vi "FindServo_NoWhile.vi"(0 "Amplitude Reference Array":refnum<vi>[](array[refnum]), 1 "Parameter Reference Arrary":refnum<vi>[](array[refnum]), 4 "Length Array":dbl[](array[numeric]), 7 "Parameter Cluster":T1={"Amplitude (cm)"=4.0, "Frequency (Hz)"=1.0, "Number of Waves"=1.0, "Length of MBE (cm)"=10.0, "Wave Exponential"=2.0, "Number of Servos"=5.0, "Bend Amplitude 1"=0.1, "Bend Amplitude 2"=0.2, "Bend Phase 1"=0.0, "Bend Phase 2"=0.8499}, 8 "Wave Form":u16(ring) items=["Sine", "Exponentional Sine", "Two Beam Bending", "Flat Plate"], 10 "2nd Mode Bending Options":u16(ring) items=["Specifiy Tail Amplitude & 1st Mode", "Specifiy Tail Amplitude & 2nd Mode", ""], 12 "Wind Up":bool, 13 "Start Time (Tick Count-millis)":u32, 14 "Wind Down":bool, 15 "Wind Down Time":i32=5, 16 "Stop In":bool, 17 "Stop Pressed Shift In (False)":bool, 19 "Ms Since Stop Shift In (Start Time)":u32, 23 "Stop In Reference":refnum<vi>, 27 "S since stop Shift In":dbl) -> (18 "Stop Out":bool, 20 "phi":dbl[](array[numeric]), 21 "X Nodes":dbl[](array[numeric]), 22 "Y Nodes":dbl[](array[numeric]), 24 "Stop Pressed Shift Out (False)":bool, 25 "MS Since Stop Shift Out":u32, 26 "S since stop Shift Out":dbl)   [LabVIEW 2017]
panel:
  out "Simulation Time":dbl
  # "Off"
  # "On"
  # "Off"
  # "On"
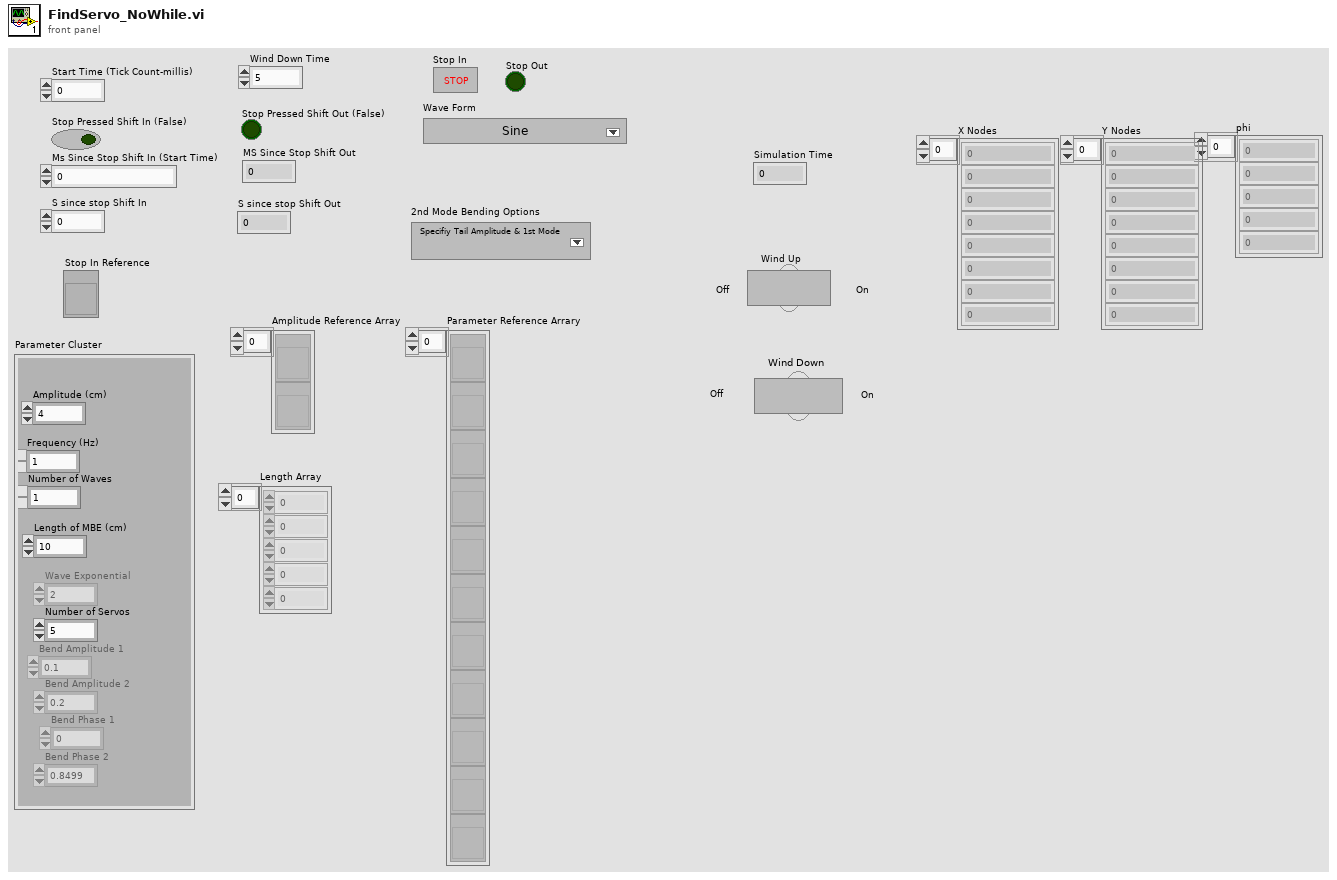
[diagram p1: front panel]
types:
  T1 = cluster{"Amplitude (cm)":dbl, "Frequency (Hz)":dbl, "Number of Waves":dbl, "Length of MBE (cm)":dbl, "Wave Exponential":dbl, "Number of Servos":dbl, "Bend Amplitude 1":dbl, "Bend Amplitude 2":dbl, "Bend Phase 1":dbl, "Bend Phase 2":dbl}
  T2 = enum8{"Enabled", "Disabled", "Disabled and Grayed Out"}
  T3 = enum8{"Enabled", "Disabled", "Disabled and Grayed Out"}[]
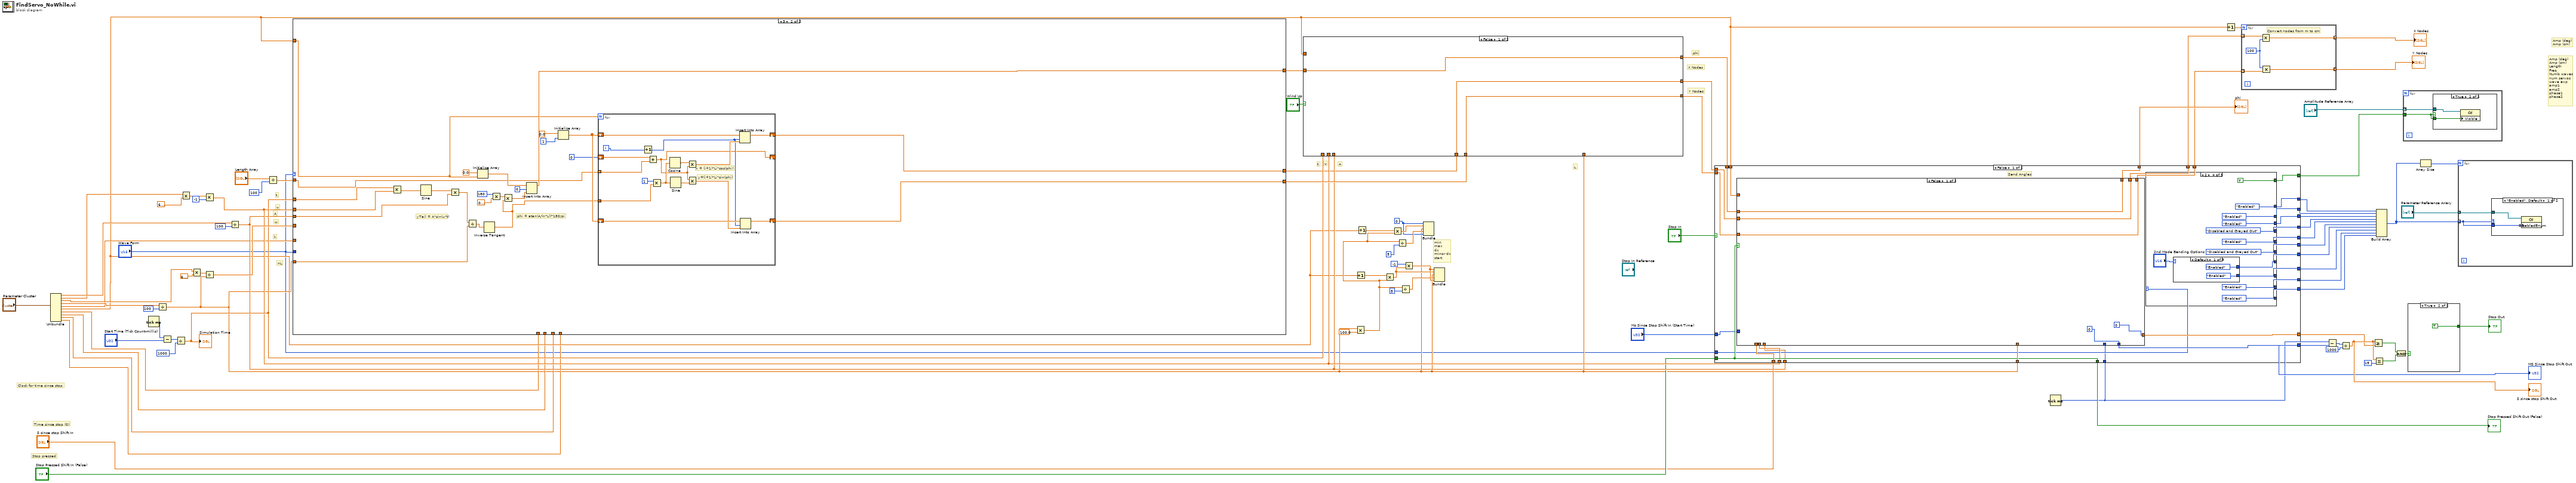
[diagram p0: block diagram]
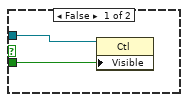
[diagram p2: hidden frame]
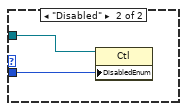
[diagram p3: hidden frame]
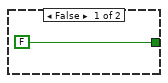
[diagram p4: hidden frame]
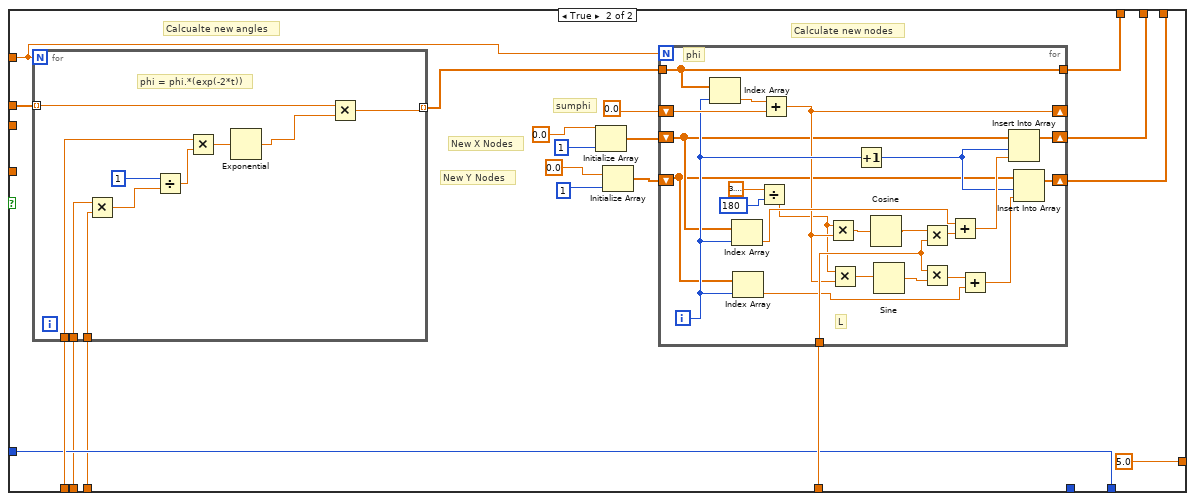
[diagram p5: hidden frame]
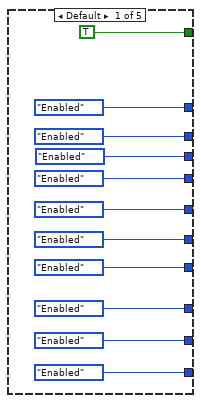
[diagram p6: hidden frame]
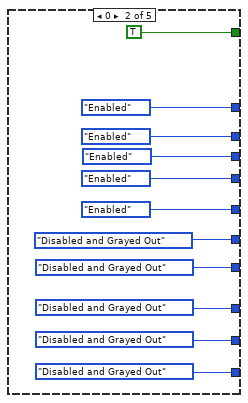
[diagram p7: hidden frame]
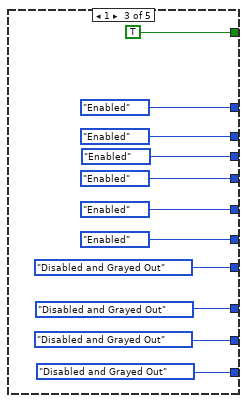
[diagram p8: hidden frame]
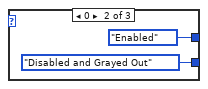
[diagram p9: hidden frame]
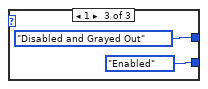
[diagram p10: hidden frame]
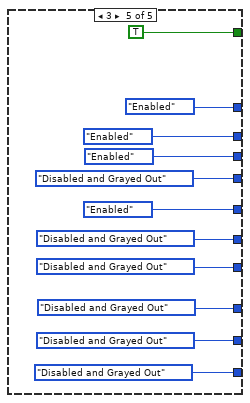
[diagram p11: hidden frame]
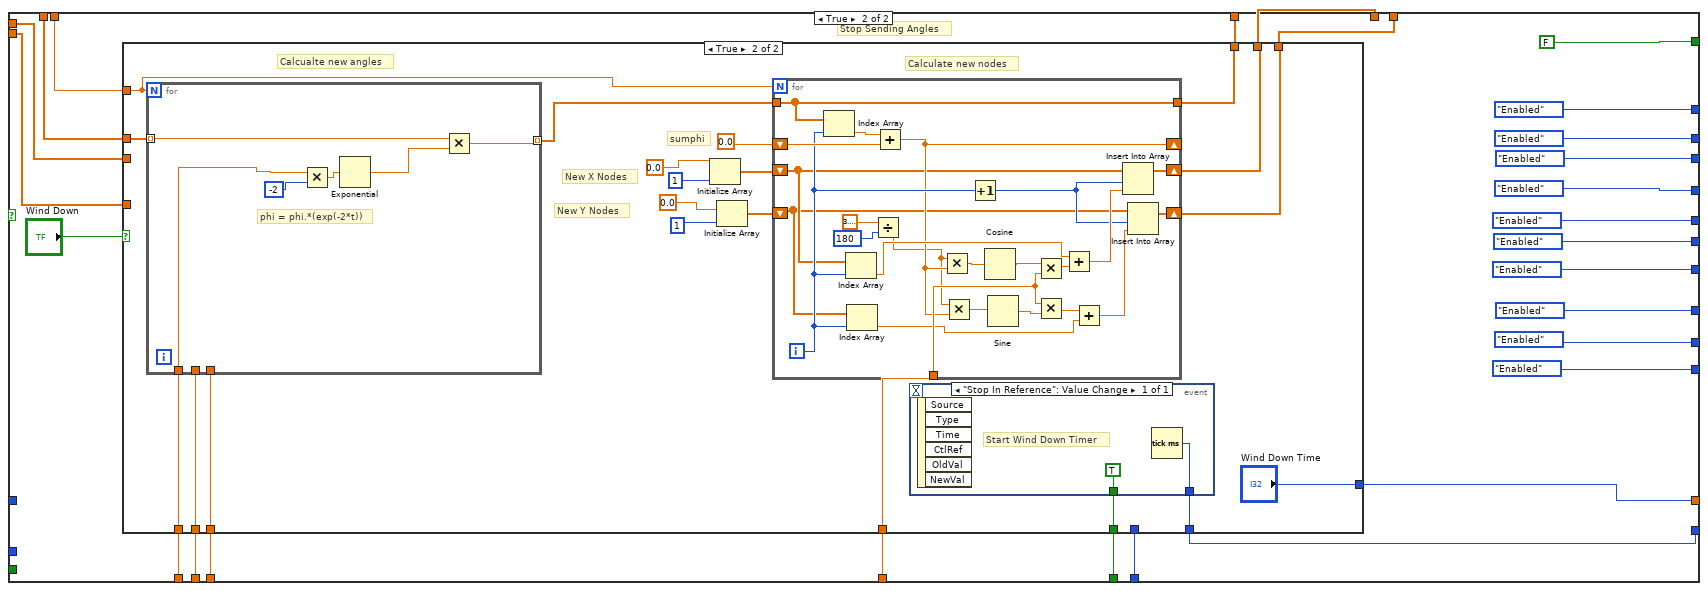
[diagram p12: hidden frame]
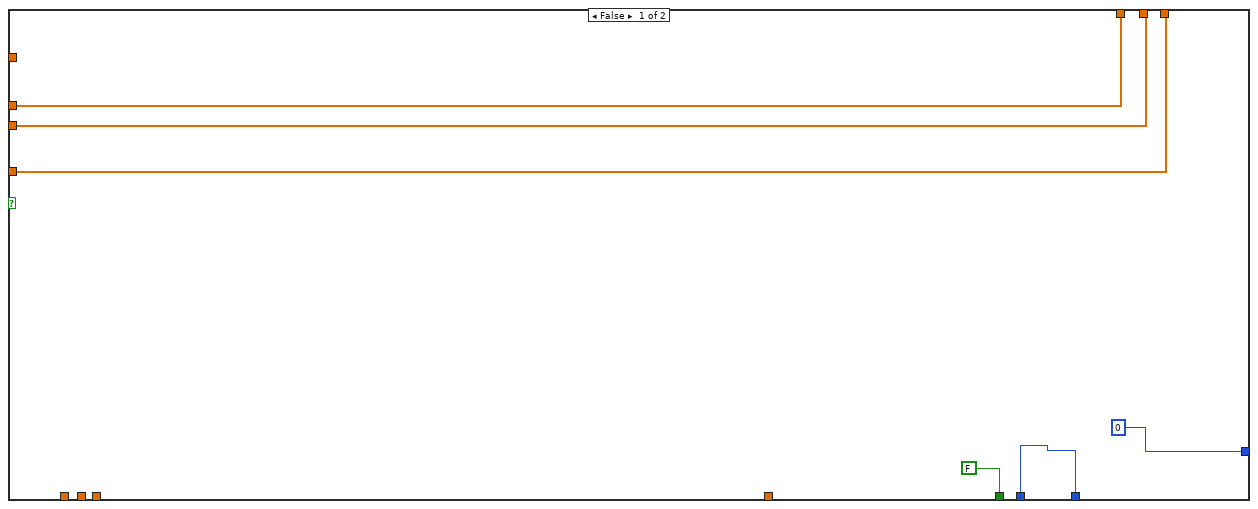
[diagram p13: hidden frame]
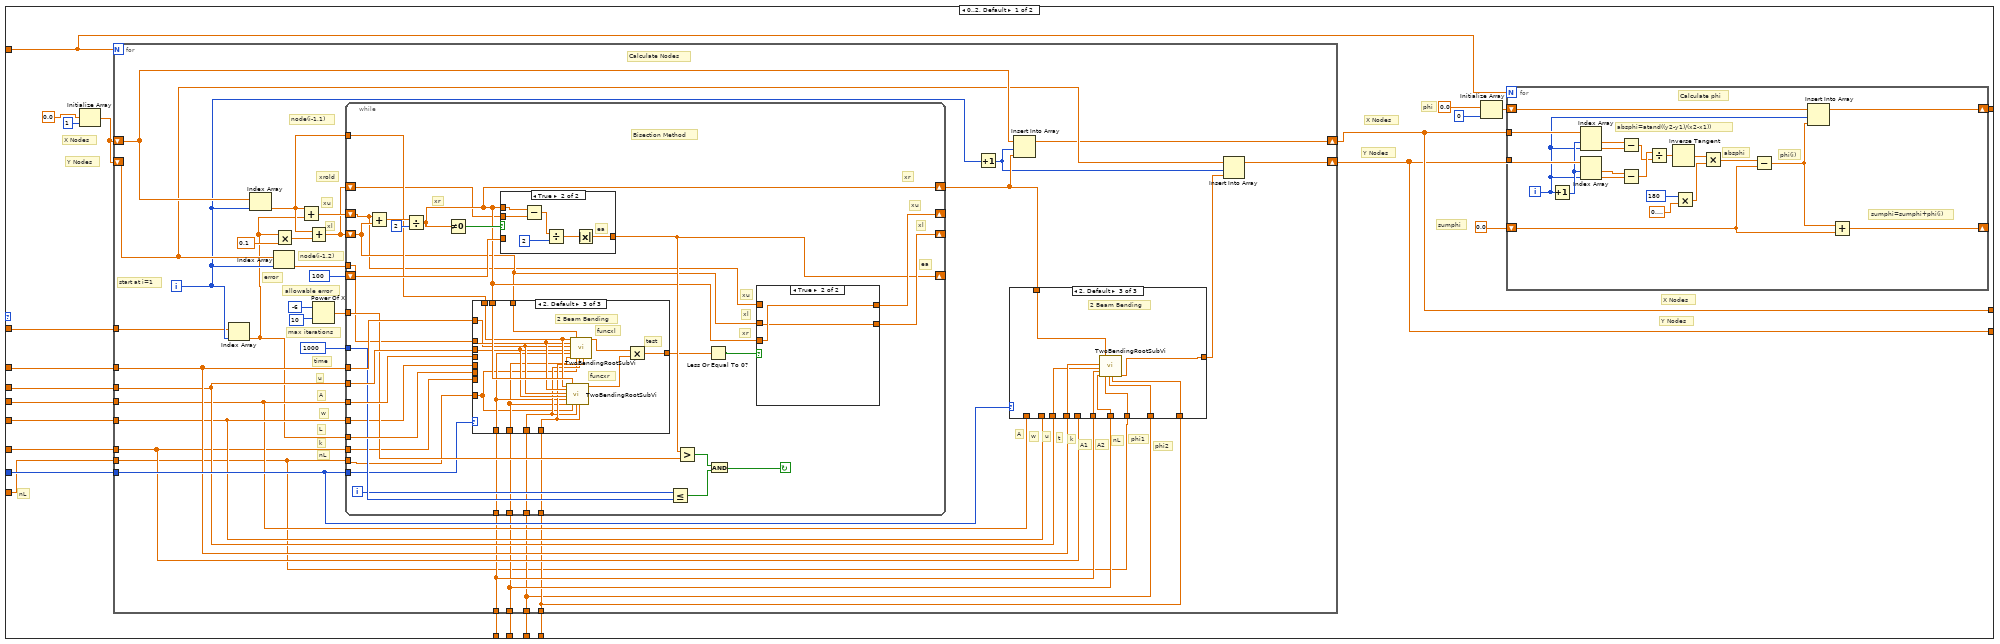
[diagram p14: hidden frame]
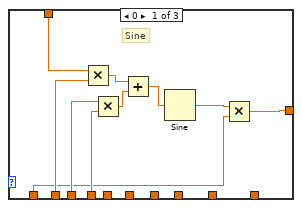
[diagram p15: hidden frame]
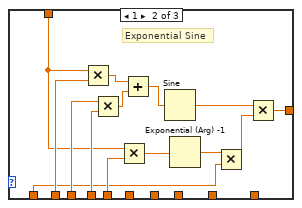
[diagram p16: hidden frame]
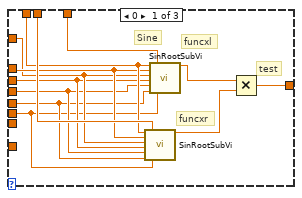
[diagram p19: hidden frame]
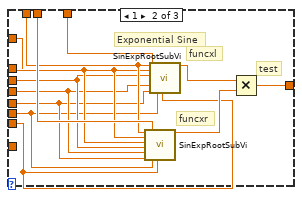
[diagram p20: hidden frame]
diagram:
  w63 = 0
  # "nL"
  # "Amp (deg)\nAmp (cm)"
  # "Amp (deg)\nAmp (cm)\nLength\nFreq\nNumb waves\nnum servos\nwave exp\namp1\namp2\nphase1\nphase2"
  # "Y Nodes"
  # "X Nodes"
  # "phi"
  # "k"
  # "min\nmax\ndx\nminor dx\nstart"
  # "A"
  # "t"
  # "L"
  # "A"
  # "u"
  # "t"
  # "u"
  # "w"
  # "Stop pressed"
  # "Clock for time since stop"
  # "Time since stop (0)"
  n1 = Unbundle("Parameter Cluster") -> ("Amplitude (cm)"=w17:dbl, "Frequency (Hz)"=w16:dbl, "Number of Waves"=w15:dbl, "Length of MBE (cm)"=w14:dbl, "Wave Exponential"=w13:dbl, "Number of Servos"=w12:dbl, "Bend Amplitude 1"=w11:dbl, "Bend Amplitude 2"=w10:dbl, "Bend Phase 1"=w9:dbl, "Bend Phase 2"=w8:dbl)
  n2 = Tick Count (ms)() -> (millisecond timer value=w78:u32)
  n3 = Divide(x=w14, y=100) -> (x/y=w3:dbl)
  n4 = Subtract(x=w78, y="Start Time (Tick Count-millis)") -> (x-y=w77:u32)
  n5 = Divide(x=w77, y=1000) -> (x/y=w59:dbl)
  "Simulation Time" <- w59
  n6 = Multiply(x=w16, y=6.283185307179586) -> (x*y=w83:dbl)
  n7 = Multiply(x=w15, y=6.283185307179586) -> (x*y=w86:dbl)
  n8 = Multiply(x=w83, y=-1) -> (x*y=w58:dbl)
  n9 = Divide(x=w86, y=w3) -> (x/y=w81:dbl)
  n10 = Divide(x=w17, y=100) -> (x/y=w57:dbl)
  n11 = Divide(x="Length Array", y=100) -> (x/y=w4:dbl[])
  n12 = case shown="3" "Wave Form" {
    tunnel: "Wave Form" -> [w111 _]
    tunnel: w81 -> [w110 _]
    tunnel: [w106 w295] -> w79
    tunnel: w57 -> [w105 w292]
    tunnel: w58 -> [w104 w304]
    tunnel: w59 -> [w103 w305]
    tunnel: [w101 w294] -> w1
    tunnel: [w100 w293] -> w75
    tunnel: w12 -> [w99 w288]
    tunnel: w13 -> [w95 _]
    tunnel: w11 -> [w94 _]
    tunnel: w10 -> [w93 _]
    tunnel: w9 -> [w92 _]
    tunnel: w8 -> [w91 _]
    tunnel: w3 -> [w90 w289]
    tunnel: w4 -> [w89 w286]
    frame 0..2, Default {
      # "nL"
      # "Y Nodes"
      # "X Nodes"
      # "Y Nodes"
      # "X Nodes"
      # "Y Nodes"
      # "X Nodes"
      # "sumphi"
      # "phi"
      n13 = Initialize Array(0.0, 1) -> (w96:dbl[])
      n14 = for {
        N: w99 -> [_]
        shift-right: [w151] -> w101
        shift-left: w96 -> [w156]
        shift-right: [w150] -> w100
        shift-left: w96 -> [w155]
        tunnel: w103 -> [w148]
        tunnel: w104 -> [w147]
        tunnel: w105 -> [w142]
        tunnel: w110 -> [w146]
        tunnel: w111 -> [w154]
        tunnel: w95 -> [w141]
        tunnel: w94 -> [w140]
        tunnel: w93 -> [w139]
        tunnel: w92 -> [w137]
        tunnel: w91 -> [w138]
        tunnel: w90 -> [w136]
        tunnel: w89 -> [w134]
        i -> [w135]
        # "nL"
        # "phi2"
        # "phi1"
        # "nL"
        # "A2"
        # "A1"
        # "k"
        # "t"
        # "u"
        # "w"
        # "A"
        # "k"
        # "Calculate Nodes"
        # "xrold"
        # "error"
        # "L"
        # "w"
        # "A"
        # "u"
        # "time"
        # "allowable error"
        # "max iterations"
        # "node(i-1,2)"
        # "node(i-1,1)"
        # "xl"
        # "xu"
        # "start at i=1"
        n15 = Index Array(array=w134, index=w135) -> (element=w133:dbl)
        n16 = Index Array(array=w156, index=w135) -> (element=w162:dbl)
        n17 = Index Array(array=w155, index=w135) -> (element=w161:dbl)
        n18 = Multiply(x=w133, y=0.1) -> (x*y=w163:dbl)
        n19 = Add(x=w162, y=w133) -> (x+y=w145:dbl)
        n20 = Add(x=w162, y=w163) -> (x+y=w144:dbl)
        n21 = Power Of X(1:10, 2:-6) -> (0:w153:dbl)
        n22 = while {
          tunnel: w162 -> [w211]
          tunnel: w161 -> [w210]
          tunnel: w153 -> [w222]
          tunnel: 1000 -> [w223]
          tunnel: w148 -> [w229]
          tunnel: w147 -> [w228]
          tunnel: w142 -> [w230]
          tunnel: w146 -> [w213]
          tunnel: w133 -> [w224]
          tunnel: w154 -> [w199]
          shift-right: [w212] -> w152
          shift-left: w144 -> [w209]
          shift-right: [w214] -> _
          shift-left: 100 -> [w225]
          shift-right: [w216] -> _
          shift-left: w145 -> [w207]
          shift-right: [w215] -> _
          shift-left: w144 -> [w208]
          tunnel: w141 -> [w204]
          tunnel: w140 -> [w203]
          tunnel: w139 -> [w202]
          tunnel: w137 -> [w201]
          tunnel: w138 -> [w200]
          tunnel: w136 -> [w198]
          i -> [w217]
          stop <- w219 continue-if-true
          # "Bisection Method"
          # "ea"
          # "xr"
          # "xu"
          # "xr"
          # "xl"
          # "xl"
          # "xu"
          # "xr"
          n23 = Add(x=w207, y=w208) -> (x+y=w227:dbl)
          n24 = Divide(x=w227, y=2) -> (x/y=w212:dbl)
          n25 = Not Equal To 0?(x=w212) -> (x != 0?=w221:bool)
          n26 = case shown="2, Default" w199 {
            tunnel: w224 -> [w245 w258 _]
            tunnel: w213 -> [w246 w259 _]
            tunnel: w230 -> [w247 w260 _]
            tunnel: w228 -> [w248 w261 w275]
            tunnel: w229 -> [w249 w262 w276]
            tunnel: w210 -> [w250 w263 w277]
            tunnel: w211 -> [w251 w264 w278]
            tunnel: w208 -> [w253 w266 w280]
            tunnel: w212 -> [w252 w265 w279]
            tunnel: [w244 w256 w272] -> w205
            tunnel: w204 -> [_ w254 _]
            tunnel: w203 -> [_ _ w269]
            tunnel: w202 -> [_ _ w268]
            tunnel: w201 -> [_ _ w270]
            tunnel: w200 -> [_ _ w271]
            tunnel: w198 -> [_ _ w267]
            frame 0 {
              # "Sine"
              # "test"
              # "funcxr"
              # "funcxl"
              n27 = call "SinRootSubVi.vi"("x node"=w251, "y node"=w250, "time"=w249, "u"=w248, "A"=w247, "w"=w246, "x"=w252, "L"=w245) -> ("SinRoot"=w243:dbl)  [unwired: 9 in, 2 out]
              n28 = call "SinRootSubVi.vi"("x node"=w251, "y node"=w250, "time"=w249, "u"=w248, "A"=w247, "w"=w246, "x"=w253, "L"=w245) -> ("SinRoot"=w242:dbl)  [unwired: 9 in, 2 out]
              n29 = Multiply(x=w242, y=w243) -> (x*y=w244:dbl)
            }
            frame 1 {
              # "Exponential Sine"
              # "test"
              # "funcxr"
              # "funcxl"
              n30 = call "SinExpRootSubVi.vi"("x node"=w264, "y node"=w263, "time"=w262, "u"=w261, "A"=w260, "w"=w259, "x"=w265, "L"=w258, "k"=w254) -> ("SinExpRoot"=w257:dbl)  [unwired: 10 in]
              n31 = call "SinExpRootSubVi.vi"("x node"=w264, "y node"=w262, "time"=w261, "u"=w266, "A"=w260, "w"=w259, "x"=w263, "L"=w258, "k"=w254) -> ("SinExpRoot"=w255:dbl)  [unwired: 10 in]
              n32 = Multiply(x=w255, y=w257) -> (x*y=w256:dbl)
            }
            frame 2, Default {
              # "2 Beam Bending"
              # "test"
              # "funcxr"
              # "funcxl"
              n33 = call "TwoBendingRootSubVi.vi"("x node"=w278, "y node"=w277, "t"=w276, "u"=w275, "amp 1"=w269, "amp 2"=w268, "x"=w279, "nL"=w267, "phi 1"=w270, "phi 2"=w271) -> ("BendRoot"=w273:dbl)  [unwired: 8 in, 1 out]
              n34 = call "TwoBendingRootSubVi.vi"("x node"=w278, "y node"=w277, "t"=w276, "u"=w275, "amp 1"=w269, "amp 2"=w268, "x"=w280, "nL"=w267, "phi 1"=w270, "phi 2"=w271) -> ("BendRoot"=w274:dbl)  [unwired: 8 in, 1 out]
              n35 = Multiply(x=w274, y=w273) -> (x*y=w272:dbl)
            }
          }
          n36 = case shown="True" w221 {
            tunnel: w225 -> [w235 _]
            tunnel: w212 -> [_ w241]
            tunnel: w209 -> [_ w240]
            tunnel: [w235 w236] -> w214
            frame False {
            }
            frame True {
              # "ea"
              n37 = Subtract(x=w241, y=w240) -> (x-y=w238:dbl)
              n38 = Divide(x=w238, y=2) -> (x/y=w237:dbl)
              n39 = Absolute Value(x=w237) -> (abs(x)=w236:dbl)
            }
          }
          n40 = Less Or Equal?(x=w217, y=w223) -> (x <= y?=w220:bool)
          n41 = Greater?(x=w214, y=w222) -> (0:w218:bool)
          n42 = Less Or Equal To 0?(x=w205) -> (x <= 0?=w206:bool)
          n43 = And(x=w218, y=w220) -> (x .and. y?=w219:bool)
          n44 = case shown="True" w206 {
            tunnel: w208 -> [_ w233]
            tunnel: w212 -> [w231 w234]
            tunnel: w207 -> [w232 _]
            tunnel: [w232 w234] -> w216
            tunnel: [w231 w233] -> w215
            frame False {
            }
            frame True {
            }
          }
        }
        n45 = Increment(x=w135) -> (x+1=w143:i32)
        n46 = case shown="2, Default" w154 {
          tunnel: [w165 w181 w197] -> w149
          tunnel: w142 -> [w166 w176 _]
          tunnel: w146 -> [w171 w186 _]
          tunnel: w147 -> [w170 w185 w194]
          tunnel: w148 -> [w169 w184 w195]
          tunnel: w152 -> [w172 w180 w196]
          tunnel: w141 -> [_ w179 _]
          tunnel: w140 -> [_ _ w191]
          tunnel: w139 -> [_ _ w190]
          tunnel: w136 -> [_ _ w189]
          tunnel: w137 -> [_ _ w193]
          tunnel: w138 -> [_ _ w192]
          frame 0 {
            # "Sine"
            n47 = Multiply(x=w172, y=w171) -> (x*y=w174:dbl)
            n48 = Multiply(x=w170, y=w169) -> (x*y=w173:dbl)
            n49 = Add(x=w174, y=w173) -> (x+y=w168:dbl)
            n50 = Sine(x=w168) -> (sin(x)=w167:dbl)
            n51 = Multiply(x=w167, y=w166) -> (x*y=w165:dbl)
          }
          frame 1 {
            # "Exponential Sine"
            n52 = Multiply(x=w180, y=w186) -> (x*y=w188:dbl)
            n53 = Multiply(x=w185, y=w184) -> (x*y=w187:dbl)
            n54 = Multiply(x=w180, y=w179) -> (x*y=w178:dbl)
            n55 = Add(x=w188, y=w187) -> (x+y=w183:dbl)
            n56 = Sine(x=w183) -> (sin(x)=w182:dbl)
            n57 = Exponential (Arg) -1(1:w178) -> (0:w177:dbl)
            n58 = Multiply(x=w177, y=w176) -> (x*y=w175:dbl)
            n59 = Multiply(x=w182, y=w175) -> (x*y=w181:dbl)
          }
          frame 2, Default {
            # "2 Beam Bending"
            n60 = call "TwoBendingRootSubVi.vi"("t"=w195, "u"=w194, "amp 1"=w191, "amp 2"=w190, "x"=w196, "nL"=w189, "phi 1"=w193, "phi 2"=w192) -> ("Bend"=w197:dbl)  [unwired: 10 in, 1 out]
          }
        }
        n61 = Insert Into Array(array=w156, index=w143, new element=w152) -> (w151:dbl[])
        n62 = Insert Into Array(array=w155, index=w143, new element=w149) -> (w150:dbl[])
      }
      n63 = Initialize Array(0.0 ("element"), 0 ("dimension size")) -> (w107:dbl[])
      n64 = for {
        N: w99 -> [_]
        tunnel: w101 -> [w120]
        tunnel: w100 -> [w132]
        shift-right: [w116] -> w106
        shift-left: w107 -> [w117]
        shift-right: [w112] -> _
        shift-left: 0.0 -> [w114]
        i -> [w118]
        # "Calculate phi"
        # "sumphi=sumphi+phi(i)"
        # "phi(i)"
        # "absphi"
        # "absphi=atand((y2-y1)/(x2-x1))"
        n65 = Increment(x=w118) -> (x+1=w119:i32)
        n66 = Index Array(array=w120, index #1=w119, index #2=w118) -> (element #1=w131:dbl, element #2=w130:dbl)
        n67 = Index Array(array=w132, index #1=w119, index #2=w118) -> (element #1=w124:dbl, element #2=w123:dbl)
        n68 = Subtract(x=w124, y=w123) -> (x-y=w129:dbl)
        n69 = Subtract(x=w131, y=w130) -> (x-y=w128:dbl)
        n70 = Divide(x=w129, y=w128) -> (x/y=w122:dbl)
        n71 = Inverse Tangent(1:w122) -> (0:w121:dbl)
        n72 = Multiply(x=180, y=0.3183098861837907) -> (x*y=w125:dbl)
        n73 = Multiply(x=w121, y=w125) -> (x*y=w115:dbl)
        n74 = Subtract(x=w115, y=w114) -> (x-y=w113:dbl)
        n75 = Insert Into Array(array=w117, index=w118, new element=w113) -> (w116:dbl[])
        n76 = Add(x=w113, y=w114) -> (x+y=w112:dbl)
      }
    }
    frame 3 {
      # "yTail = A*sin(u*t)"
      # "phi = atan(A/(n*L))*180/pi"
      n77 = Multiply(x=w305, y=w304) -> (x*y=w303:dbl)
      n78 = Sine(x=w303) -> (sin(x)=w302:dbl)
      n79 = Multiply(x=w302, y=w292) -> (x*y=w291:dbl)
      n80 = Divide(x=w291, y=w289) -> (x/y=w290:dbl)
      n81 = Initialize Array(0.0, w288) -> (w300:dbl[])
      n82 = Inverse Tangent(1:w290) -> (0:w284:dbl)
      n83 = Multiply(x=180, y=0.3183098861837907) -> (x*y=w283:dbl)
      n84 = Multiply(x=w283, y=w284) -> (x*y=w285:dbl)
      n85 = Insert Into Array(array=w300, index=0, new element=w285) -> (w295:dbl[])
      n86 = Initialize Array(0.0 ("element"), 1 ("dimension size")) -> (w296:dbl[])
      n87 = for {
        N: w288 -> [_]
        tunnel: w286 -> [w307] mode=indexing
        tunnel: w284 -> [w319]
        shift-right: [w316] -> w294
        shift-left: w296 -> [w317]
        shift-right: [w313] -> w293
        shift-left: w296 -> [w314]
        shift-right: [w306] -> _
        shift-left: 0 -> [w308]
        i -> [w309]
        # "y=(i+1)*Li*sin(phi)"
        # "x = (i+1)*Li*cos(phi)"
        n88 = Increment(x=w309) -> (x+1=w311:i32)
        n89 = Add(x=w308, y=w307) -> (x+y=w306:dbl)
        n90 = Multiply(x=1, y=w319) -> (x*y=w318:dbl)
        n91 = Cosine(x=w318) -> (cos(x)=w321:dbl)
        n92 = Sine(x=w318) -> (sin(x)=w320:dbl)
        n93 = Multiply(x=w321, y=w306) -> (x*y=w315:dbl)
        n94 = Multiply(x=w306, y=w320) -> (x*y=w312:dbl)
        n95 = Insert Into Array(array=w317, index=w311, new element=w315) -> (w316:dbl[])
        n96 = Insert Into Array(array=w314, index=w311, new element=w312) -> (w313:dbl[])
      }
    }
  }
  n97 = case shown="False" "Wind Up" {
    tunnel: w79 -> [w324 w341]
    tunnel: [w324 w337] -> w60
    tunnel: w12 -> [_ w333]
    tunnel: w57 -> [_ w340]
    tunnel: w58 -> [_ w339]
    tunnel: w59 -> [_ w338]
    tunnel: [w323 w332] -> w56
    tunnel: [w322 w331] -> w55
    tunnel: w3 -> [_ w335]
    tunnel: w1 -> [w323 _]
    tunnel: w75 -> [w322 _]
    frame False {
    }
    frame True {
      # "New X Nodes"
      # "New Y Nodes"
      # "sumphi"
      n98 = for {
        N: w333 -> [_]
        tunnel: w341 -> [w370] mode=indexing
        tunnel: [w369] -> w334 mode=indexing
        tunnel: w340 -> [w377]
        tunnel: w339 -> [w376]
        tunnel: w338 -> [w374]
        # "Calcualte new angles"
        # "phi = phi.*(1-exp(t/(u*A)))"
        n99 = Multiply(x=w376, y=w377) -> (x*y=w375:dbl)
        n100 = Divide(x=w374, y=w375) -> (x/y=w367:dbl)
        n101 = Multiply(x=w367, y=0.5) -> (x*y=w368:dbl)
        n102 = Exponential(1:w368) -> (0:w373:dbl)
        n103 = Subtract(x=1, y=w373) -> (x-y=w371:dbl)
        n104 = Multiply(x=w370, y=w371) -> (x*y=w369:dbl)
      }
      n105 = Initialize Array(0.0 ("element"), 1 ("dimension size")) -> (w326:dbl[])
      n106 = Initialize Array(0.0 ("element"), 1 ("dimension size")) -> (w325:dbl[])
      n107 = for {
        N: w333 -> [_]
        shift-right: [w345] -> _
        shift-left: 0.0 -> [w365]
        tunnel: w334 -> [w364]
        tunnel: [w364] -> w337
        tunnel: w335 -> [w362]
        shift-right: [w355] -> w332
        shift-left: w326 -> [w343]
        shift-right: [w354] -> w331
        shift-left: w325 -> [w342]
        i -> [w353]
        # "Calculate new nodes"
        n108 = Index Array(array=w364, index=w353) -> (element=w363:dbl)
        n109 = Index Array(array=w343, index=w353) -> (element=w361:dbl)
        n110 = Index Array(array=w342, index=w353) -> (element=w358:dbl)
        n111 = Divide(x=3.141592653589793, y=180) -> (x/y=w344:dbl)
        n112 = Add(x=w363, y=w365) -> (x+y=w345:dbl)
        n113 = Multiply(x=w344, y=w345) -> (x*y=w347:dbl)
        n114 = Multiply(x=w344, y=w345) -> (x*y=w346:dbl)
        n115 = Increment(x=w353) -> (x+1=w352:i32)
        n116 = Cosine(x=w347) -> (cos(x)=w351:dbl)
        n117 = Sine(x=w346) -> (sin(x)=w350:dbl)
        n118 = Multiply(x=w351, y=w362) -> (x*y=w360:dbl)
        n119 = Multiply(x=w362, y=w350) -> (x*y=w359:dbl)
        n120 = Add(x=w361, y=w360) -> (x+y=w357:dbl)
        n121 = Add(x=w359, y=w358) -> (x+y=w356:dbl)
        n122 = Insert Into Array(array=w343, index=w352, new element=w357) -> (w355:dbl[])
        n123 = Insert Into Array(array=w342, index=w352, new element=w356) -> (w354:dbl[])
      }
    }
  }
  n124 = Multiply(x=w3, y=100.0) -> (x*y=w61:dbl)
  n125 = Increment(x=w12) -> (x+1=w73:dbl)
  n126 = Increment(x=w12) -> (x+1=w70:dbl)
  n127 = Multiply(x=w73, y=w61) -> (x*y=w71:dbl)
  n128 = Multiply(x=w70, y=w61) -> (x*y=w67:dbl)
  n129 = Divide(x=w61, y=5) -> (x/y=w68:dbl)
  n130 = Divide(x=w61, y=5) -> (x/y=w69:dbl)
  n131 = Multiply(x=-1, y=w71) -> (x*y=w72:dbl)
  n132 = Bundle(w63, w67, w3, w68, w63) -> ()  [unwired: 1 in, 1 out]
  n133 = Bundle(w72, w71, w3, w69, w72) -> ()  [unwired: 1 in, 1 out]
  n134 = Tick Count (ms)() -> (millisecond timer value=w42:u32)
  n135 = case shown="False" "Stop In" {
    tunnel: "Wave Form" -> [w382 _]
    tunnel: [w378 FALSE] -> w7
    tunnel: [w405 T2."Enabled" ("Disabled")] -> w23
    tunnel: [w404 T2."Enabled" ("Disabled")] -> w34
    tunnel: [w396 T2."Enabled" ("Disabled")] -> w33
    tunnel: [w403 T2."Enabled" ("Disabled")] -> w32
    tunnel: [w402 T2."Enabled" ("Disabled")] -> w31
    tunnel: [w401 T2."Enabled" ("Disabled")] -> w30
    tunnel: [w400 T2."Enabled" ("Disabled")] -> w29
    tunnel: [w399 T2."Enabled" ("Disabled")] -> w28
    tunnel: [w398 T2."Enabled" ("Disabled")] -> w27
    tunnel: [w397 T2."Enabled" ("Disabled")] -> w26
    tunnel: w12 -> [w393 w540]
    tunnel: w60 -> [w390 w539]
    tunnel: w3 -> [w395 w538]
    tunnel: "S since stop Shift In" -> [w394 w537]
    tunnel: w58 -> [w383 w536]
    tunnel: w57 -> [w381 w535]
    tunnel: w56 -> [w389 w534]
    tunnel: w55 -> [w388 w533]
    tunnel: [w379 w530] -> w54
    tunnel: [w391 w529] -> w53
    tunnel: [w392 w528] -> w36
    tunnel: "Stop Pressed Shift In (False)" -> [w387 _]
    tunnel: [w387 w532] -> w48
    tunnel: [w384 w531] -> w47
    tunnel: "Ms Since Stop Shift In (Start Time)" -> [w386 _]
    tunnel: [w385 w527] -> w46
    tunnel: w42 -> [w380 w526]
    frame False {
      # "Send Angles"
      n136 = case shown="False" w387 {
        tunnel: w390 -> [w410 w429]
        tunnel: [w410 w427] -> w379
        tunnel: w393 -> [_ w423]
        tunnel: w394 -> [_ w428]
        tunnel: [w409 w422] -> w391
        tunnel: [w408 w421] -> w392
        tunnel: w395 -> [_ w425]
        tunnel: w389 -> [w409 _]
        tunnel: w388 -> [w408 _]
        tunnel: [0 w414] -> w384
        tunnel: w386 -> [_ w414]
        tunnel: [0 5.0] -> w385
        tunnel: w383 -> [_ w412]
        tunnel: w381 -> [_ w411]
        tunnel: w380 -> [_ _]
        frame False {
        }
        frame True {
          # "New X Nodes"
          # "New Y Nodes"
          # "sumphi"
          # "Calculate new nodes"
          # "Calcualte new angles"
          n137 = for {
            N: w423 -> [_]
            tunnel: w429 -> [w463] mode=indexing
            tunnel: [w462] -> w424 mode=indexing
            tunnel: w428 -> [w461]
            tunnel: w412 -> [w457]
            tunnel: w411 -> [w458]
            # "phi = phi.*(exp(-2*t))"
            n138 = Multiply(x=w457, y=w458) -> (x*y=w456:dbl)
            n139 = Divide(x=1, y=w456) -> (x/y=w454:dbl)
            n140 = Multiply(x=w461, y=w454) -> (x*y=w460:dbl)
            n141 = Exponential(1:w460) -> (0:w459:dbl)
            n142 = Multiply(x=w463, y=w459) -> (x*y=w462:dbl)
          }
          n143 = Initialize Array(0.0 ("element"), 1 ("dimension size")) -> (w416:dbl[])
          n144 = Initialize Array(0.0 ("element"), 1 ("dimension size")) -> (w415:dbl[])
          n145 = for {
            N: w423 -> [_]
            shift-right: [w433] -> _
            shift-left: 0.0 -> [w453]
            tunnel: w424 -> [w452]
            tunnel: [w452] -> w427
            tunnel: w425 -> [w450]
            shift-right: [w443] -> w422
            shift-left: w416 -> [w431]
            shift-right: [w442] -> w421
            shift-left: w415 -> [w430]
            i -> [w441]
            # "phi"
            # "L"
            n146 = Index Array(array=w452, index=w441) -> (element=w451:dbl)
            n147 = Index Array(array=w431, index=w441) -> (element=w449:dbl)
            n148 = Index Array(array=w430, index=w441) -> (element=w446:dbl)
            n149 = Divide(x=3.141592653589793, y=180) -> (x/y=w432:dbl)
            n150 = Add(x=w451, y=w453) -> (x+y=w433:dbl)
            n151 = Multiply(x=w432, y=w433) -> (x*y=w435:dbl)
            n152 = Multiply(x=w432, y=w433) -> (x*y=w434:dbl)
            n153 = Increment(x=w441) -> (x+1=w440:i32)
            n154 = Cosine(x=w435) -> (cos(x)=w439:dbl)
            n155 = Sine(x=w434) -> (sin(x)=w438:dbl)
            n156 = Multiply(x=w439, y=w450) -> (x*y=w448:dbl)
            n157 = Multiply(x=w450, y=w438) -> (x*y=w447:dbl)
            n158 = Add(x=w449, y=w448) -> (x+y=w445:dbl)
            n159 = Add(x=w447, y=w446) -> (x+y=w444:dbl)
            n160 = Insert Into Array(array=w431, index=w440, new element=w445) -> (w443:dbl[])
            n161 = Insert Into Array(array=w430, index=w440, new element=w444) -> (w442:dbl[])
          }
        }
      }
      n162 = case shown="2" w382 {
        tunnel: [TRUE TRUE TRUE TRUE TRUE] -> w378
        tunnel: [T2."Enabled" ("Disabled") T2."Enabled" ("Disabled") T2."Enabled" ("Disabled") T2."Enabled" ("Disabled") T2."Enabled" ("Disabled")] -> w405
        tunnel: [T2."Enabled" ("Disabled") T2."Enabled" ("Disabled") T2."Enabled" ("Disabled") T2."Enabled" ("Disabled") T2."Enabled" ("Disabled")] -> w404
        tunnel: [T2."Enabled" ("Disabled") T2."Enabled" ("Disabled") T2."Enabled" ("Disabled") T2."Enabled" ("Disabled") T2."Enabled" ("Disabled")] -> w396
        tunnel: [T2."Enabled" ("Disabled") T2."Enabled" ("Disabled") T2."Enabled" ("Disabled") T2."Disabled and Grayed Out" ("Disabled") T2."Disabled and Grayed Out" ("Disabled")] -> w403
        tunnel: [T2."Enabled" ("Disabled") T2."Enabled" ("Disabled") T2."Enabled" ("Disabled") T2."Enabled" ("Disabled") T2."Enabled" ("Disabled")] -> w402
        tunnel: [T2."Enabled" ("Disabled") T2."Disabled and Grayed Out" ("Disabled") T2."Enabled" ("Disabled") T2."Disabled and Grayed Out" ("Disabled") T2."Disabled and Grayed Out" ("Disabled")] -> w401
        tunnel: [T2."Enabled" ("Disabled") T2."Disabled and Grayed Out" ("Disabled") T2."Disabled and Grayed Out" ("Disabled") w498 T2."Disabled and Grayed Out" ("Disabled")] -> w400
        tunnel: [T2."Enabled" ("Disabled") T2."Disabled and Grayed Out" ("Disabled") T2."Disabled and Grayed Out" ("Disabled") w497 T2."Disabled and Grayed Out" ("Disabled")] -> w399
        tunnel: [T2."Enabled" ("Disabled") T2."Disabled and Grayed Out" ("Disabled") T2."Disabled and Grayed Out" ("Disabled") T2."Enabled" ("Disabled") T2."Disabled and Grayed Out" ("Disabled")] -> w398
        tunnel: [T2."Enabled" ("Disabled") T2."Disabled and Grayed Out" ("Disabled") T2."Disabled and Grayed Out" ("Disabled") T2."Enabled" ("Disabled") T2."Disabled and Grayed Out" ("Disabled")] -> w397
        frame Default {
        }
        frame 0 {
        }
        frame 1 {
        }
        frame 2 {
          n163 = case shown="Default" "2nd Mode Bending Options" {
            tunnel: [T2."Enabled" ("Disabled") T2."Enabled" ("Disabled") T2."Disabled and Grayed Out" ("Disabled")] -> w498
            tunnel: [T2."Enabled" ("Disabled") T2."Disabled and Grayed Out" ("Disabled") T2."Enabled" ("Disabled")] -> w497
            frame Default {
            }
            frame 0 {
            }
            frame 1 {
            }
          }
        }
        frame 3 {
        }
      }
    }
    frame True {
      # "Stop Sending Angles"
      n164 = case shown="True" "Wind Down" {
        tunnel: w539 -> [w558 w578]
        tunnel: [w558 w574] -> w530
        tunnel: w540 -> [_ w570]
        tunnel: w535 -> [_ w577]
        tunnel: w536 -> [_ w576]
        tunnel: w537 -> [_ w575]
        tunnel: [w557 w569] -> w529
        tunnel: [w556 w568] -> w528
        tunnel: w538 -> [_ w572]
        tunnel: w534 -> [w557 _]
        tunnel: w533 -> [w556 _]
        tunnel: [FALSE w561] -> w532
        tunnel: [0 "Wind Down Time"] -> w527
        tunnel: [w553 w560] -> w531
        tunnel: w526 -> [w553 _]
        frame False {
        }
        frame True {
          # "New X Nodes"
          # "New Y Nodes"
          # "sumphi"
          # "Calculate new nodes"
          # "Calcualte new angles"
          n165 = for {
            N: w570 -> [_]
            tunnel: w578 -> [w610] mode=indexing
            tunnel: [w609] -> w571 mode=indexing
            tunnel: w577 -> [_]
            tunnel: w576 -> [_]
            tunnel: w575 -> [w605]
            # "phi = phi.*(exp(-2*t))"
            n166 = Multiply(x=w605, y=-2) -> (x*y=w606:dbl)
            n167 = Exponential(1:w606) -> (0:w607:dbl)
            n168 = Multiply(x=w610, y=w607) -> (x*y=w609:dbl)
          }
          n169 = Initialize Array(0.0 ("element"), 1 ("dimension size")) -> (w563:dbl[])
          n170 = Initialize Array(0.0 ("element"), 1 ("dimension size")) -> (w562:dbl[])
          n171 = for {
            N: w570 -> [_]
            shift-right: [w584] -> _
            shift-left: 0.0 -> [w604]
            tunnel: w571 -> [w603]
            tunnel: [w603] -> w574
            tunnel: w572 -> [w601]
            shift-right: [w594] -> w569
            shift-left: w563 -> [w582]
            shift-right: [w593] -> w568
            shift-left: w562 -> [w581]
            i -> [w592]
            n172 = Index Array(array=w603, index=w592) -> (element=w602:dbl)
            n173 = Index Array(array=w582, index=w592) -> (element=w600:dbl)
            n174 = Index Array(array=w581, index=w592) -> (element=w597:dbl)
            n175 = Divide(x=3.141592653589793, y=180) -> (x/y=w583:dbl)
            n176 = Add(x=w602, y=w604) -> (x+y=w584:dbl)
            n177 = Multiply(x=w583, y=w584) -> (x*y=w586:dbl)
            n178 = Multiply(x=w583, y=w584) -> (x*y=w585:dbl)
            n179 = Increment(x=w592) -> (x+1=w591:i32)
            n180 = Cosine(x=w586) -> (cos(x)=w590:dbl)
            n181 = Sine(x=w585) -> (sin(x)=w589:dbl)
            n182 = Multiply(x=w590, y=w601) -> (x*y=w599:dbl)
            n183 = Multiply(x=w601, y=w589) -> (x*y=w598:dbl)
            n184 = Add(x=w600, y=w599) -> (x+y=w596:dbl)
            n185 = Add(x=w598, y=w597) -> (x+y=w595:dbl)
            n186 = Insert Into Array(array=w582, index=w591, new element=w596) -> (w594:dbl[])
            n187 = Insert Into Array(array=w581, index=w591, new element=w595) -> (w593:dbl[])
          }
          n188 = event shown="[0] \"Stop In Reference\": Value Change" {
            selector: _ -> [_]
            dyn-events: _ -> [_]
            timeout: _ -> [_]
            tunnel: [TRUE] -> w561
            tunnel: [w579] -> w560
            event "Stop In Reference": Value Change {
              # "Start Wind Down Timer"
              n189 = event-data() -> ()  [unwired: 1 in, 6 out]
              n190 = Tick Count (ms)() -> (millisecond timer value=w579:u32)
            }
          }
        }
      }
    }
  }
  "phi" <- w54
  "Stop Pressed Shift Out (False)" <- w48
  "MS Since Stop Shift Out" <- w47
  n191 = Increment(x=w12) -> (x+1=w74:dbl)
  n192 = for {
    N: w74 -> [_]
    tunnel: w53 -> [w615] mode=indexing
    tunnel: w36 -> [w613] mode=indexing
    tunnel: [w612] -> w37 mode=indexing
    tunnel: [w611] -> w35 mode=indexing
    w614 = 100
    # "Convert nodes from m to cm"
    n193 = Multiply(x=w615, y=w614) -> (x*y=w612:dbl)
    n194 = Multiply(x=w614, y=w613) -> (x*y=w611:dbl)
  }
  "X Nodes" <- w37
  "Y Nodes" <- w35
  n195 = Subtract(x=w42, y=w47) -> (x-y=w50:u32)
  n196 = Divide(x=w50, y=1000) -> (x/y=w49:dbl)
  "S since stop Shift Out" <- w49
  n197 = Greater Or Equal?(x=w49, y=w46) -> (x >= y?=w44:bool)
  n198 = Less Or Equal?(x=w49, y=15) -> (x <= y?=w43:bool)
  n199 = Build Array(w23, w34, w33, w32, w31, w30, w29, w28, w27, w26) -> (w24:T3)
  n200 = And(x=w44, y=w43) -> (x .and. y?=w45:bool)
  n201 = for {
    tunnel: w7 -> [w616]
    tunnel: "Amplitude Reference Array" -> [w617] mode=indexing
    n202 = case shown="True" w616 {
      tunnel: w617 -> [w618 w621]
      tunnel: w616 -> [w619 w620]
      frame False {
        n203 = property on="Property Node" class="Ctl"(reference=w618, "Visible"=w619) -> ()  [unwired: 1 in, 2 out]
      }
      frame True {
        n204 = property on="Property Node" class="Ctl"(reference=w621, "Visible"=w620) -> ()  [unwired: 1 in, 2 out]
      }
    }
  }
  n205 = case shown="True" w45 {
    tunnel: [FALSE TRUE] -> w41
    frame False {
    }
    frame True {
    }
  }
  "Stop Out" <- w41
  n206 = Array Size(array=w24) -> (size(s)=w25:i32)
  n207 = for {
    N: w25 -> [_]
    tunnel: w24 -> [w625] mode=indexing
    tunnel: "Parameter Reference Arrary" -> [w624] mode=indexing
    n208 = case shown="\"Enabled\", Default" w625 {
      tunnel: w625 -> [w627 w629]
      tunnel: w624 -> [w626 w628]
      frame "Enabled", Default {
        n209 = property on="Property Node" class="Ctl"(reference=w626, "DisabledEnum"=w627) -> ()  [unwired: 1 in, 2 out]
      }
      frame "Disabled" {
        n210 = property on="Property Node" class="Ctl"(reference=w628, "DisabledEnum"=w629) -> ()  [unwired: 1 in, 2 out]
      }
    }
  }
